vi "Timestamp.vi"(11 "Semiconductor Module Context":T1) -> (0 "error out":errorcluster, 2 "Time In Double":dbl, 3 "current time 2":timestamp)   [LabVIEW 2013]
uses:
  <vilib>/NI_TestStand_SemiconductorModule/NI_TestStand_Semiconductor_Module.lvlibp/PinMap/General/SemiconductorModuleContext.ctl
  <vilib>/NI_TestStand_SemiconductorModule/NI_TestStand_Semiconductor_Module.lvlibp/PinMap/DC Power/PinToNIDCPowerSession.vi
  <vilib>/NI_TestStand_SemiconductorModule/NI_TestStand_Semiconductor_Module.lvlibp/PinMap/Deprecated/PublishDataDoubleSinglePinSingleInstrument.vi
  <vilib>/NI_TestStand_SemiconductorModule/NI_TestStand_Semiconductor_Module.lvlibp
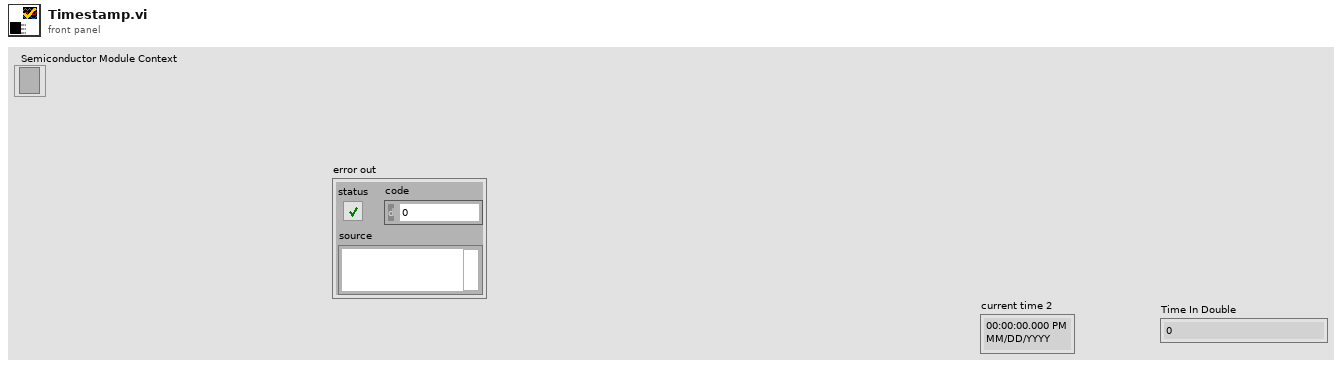
[diagram p1: front panel]
types:
  T1 = typedef "NI_TestStand_Semiconductor_Module.lvlibp/SemiconductorModuleContext.ctl" = refnum<k7>
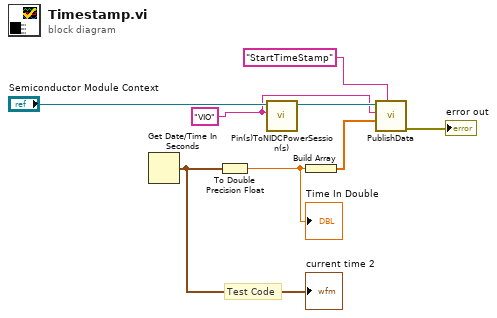
[diagram p0: block diagram]
diagram:
  w1 = "VIO" ("Pin")
  # "Test Code"
  n1 = Get Date/Time In Seconds() -> (seconds since 1Jan1904=w8:timestamp)
  "current time 2" <- w8
  n2 = To Double Precision Float(number=w8) -> (double precision float=w5:dbl)
  "Time In Double" <- w5
  n3 = call-poly <vilib>:"Pin(s)ToNIDCPowerSession(s).vi"("Pin"=w1, "Semiconductor Module Context"="Semiconductor Module Context") -> ("Semiconductor Module Context Out"=w6:T1)  [unwired: 5 in, 4 out]
  n4 = Build Array(w5) -> (w4:dbl[])
  n5 = call-poly <vilib>:"PublishData.vi"("Measurement Id"="StartTimeStamp", "Data In"=w4, "Pin"=w1, "Semiconductor Module Context"=w6) -> ("error out"=→"error out":errorcluster)  [unwired: 6 in, 1 out]
